vi "VR-Hall.vi"(8 "error in (no error)":errorcluster, 11 "Node Ptr":T2 format="%.0x") -> (0 "error out":errorcluster)   [LabVIEW 2016, in "DCM System Explorer.lvlib"]
uses:
  DCM System Explorer.lvlib
  <vilib>/NI Veristand/Custom Device API/Custom Device Item Ref.ctl
  <vilib>/Powertrain Controls/Device Drivers/VR-Hall/RevC/Real-Time/Support/Vr_Hall_mode_control_revc.ctl
  Shared/DCM Properties.vi
  <vilib>/NI Veristand/Custom Device API/Get Item Property (Double Array).vi
  <vilib>/NI Veristand/Custom Device API/Set Item Property (Double Array).vi
  <vilib>/NI VeriStand/Custom Device API/Custom Device API.lvlib
  DCM Shared.lvlib
panel:
  out "Channel":string[](array[string])=["Channel 1", "Channel 2", "Channel 3", "Channel 4", "Channel 5"]
  in  "Arming Threshold [V]":dbl[](array[numeric])
  in  "VR-Hall Mode Select":T1[](array[typedef])
  in  "Header":cluster{"Section Name":string}={"Section Name"="VR-Hall Initial Settings"}
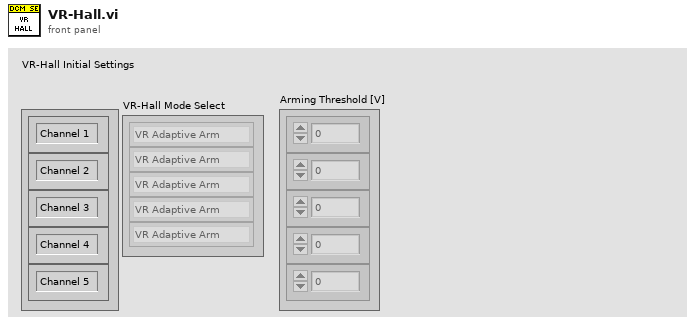
[diagram p1: front panel]
types:
  T1 = typedef "Vr_Hall_mode_control_revc.ctl" = enum32{"VR Adaptive Arm", "VR Manual Arm", "Hall", "Hall w/ Pull-up"}
  T2 = typedef "Custom Device API.lvlib/Custom Device Item Ref.ctl" = u64
  T3 = typedef "Custom Device API.lvlib/Custom Device Commands.ctl" = enum16{"Default", "Item renamed", "Shutdown", "Dynamic button pressed"}
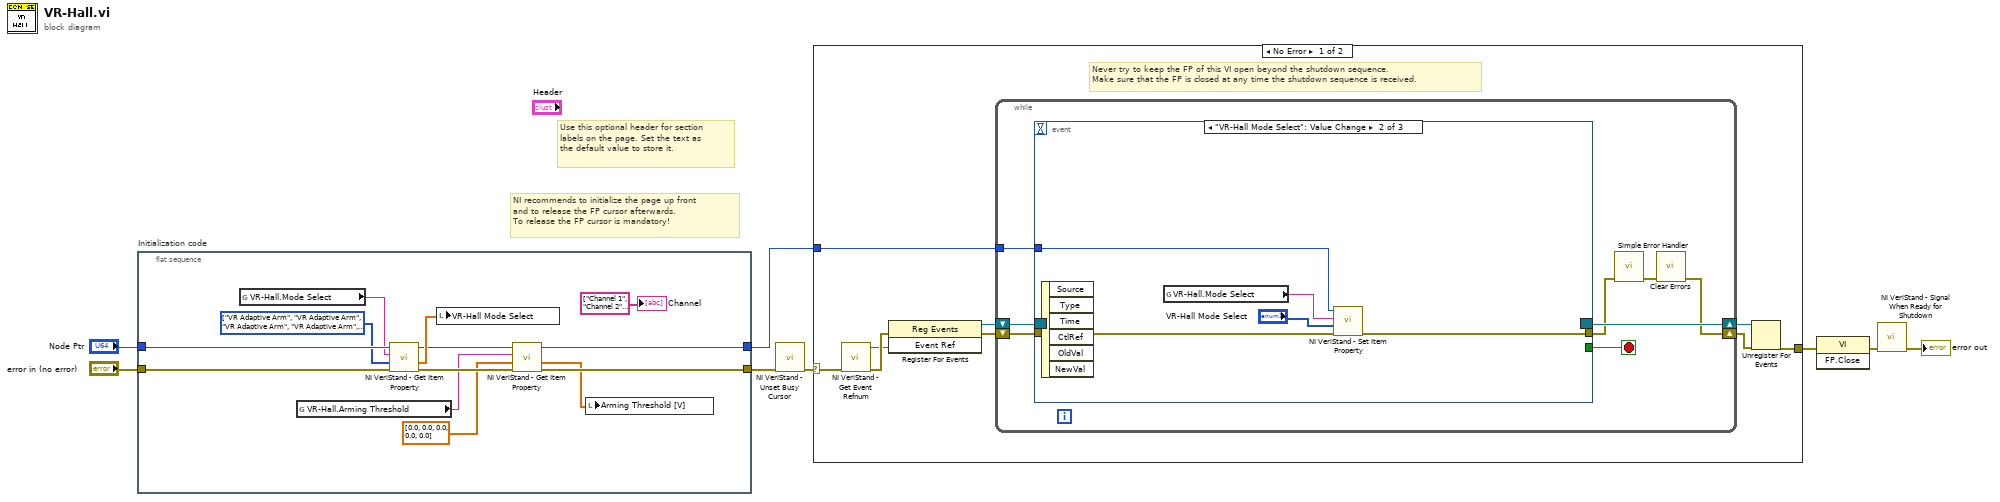
[diagram p0: block diagram]
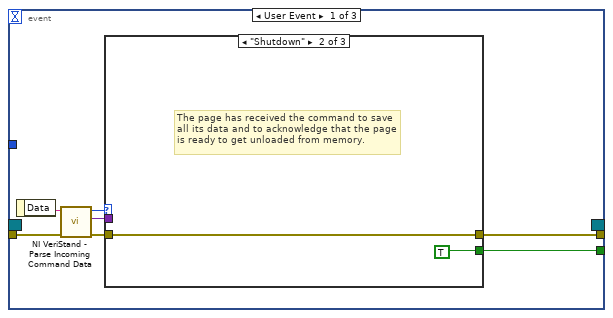
[diagram p2: hidden frame]
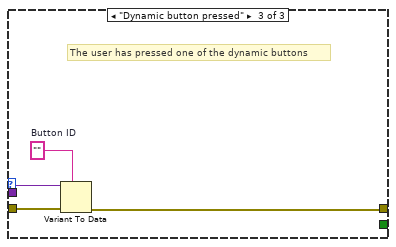
[diagram p4: hidden frame]
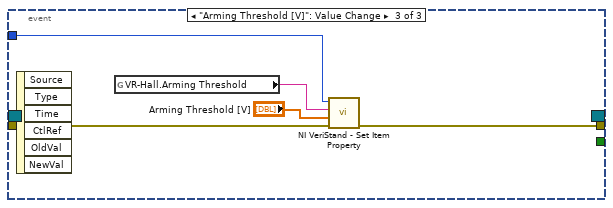
[diagram p5: hidden frame]
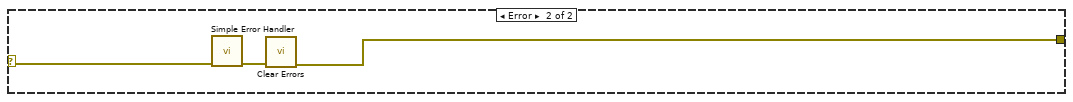
[diagram p6: hidden frame]
diagram:
  # "Use this optional header for section labels on the page. Set the text as the default value to store it."
  # "NI recommends to initialize the page up front\nand to release the FP cursor afterwards.\nTo release the FP cursor is mandatory!"
  n1 = flat-sequence "Initialization code" {
    tunnel: "error in (no error)" -> [w19]
    tunnel: "Node Ptr" -> [w20]
    tunnel: [w13] -> w4
    tunnel: [w14] -> w1
    frame #0 {
      w17 = T1[] [enum."VR Adaptive Arm", enum."VR Adaptive Arm", enum."VR Adaptive Arm", enum."VR Adaptive Arm", enum."VR Adaptive Arm"] items=["VR Adaptive Arm", "VR Manual Arm", "Hall", "Hall w/ Pull-up"] ("VR-Hall Mode Select")
      n2 = global read "DCM Properties.vi" "VR-Hall.Mode Select"() -> (w18:string)
      n3 = global read "DCM Properties.vi" "VR-Hall.Arming Threshold"() -> (w11:string)
      n4 = call-poly <vilib>:"NI VeriStand - Get Item Property.vi"("error in (no error)"=w19, "Default Value"=w17, "Property Name"=w18, "Item Ref in"=w20) -> ("error out"=w12:errorcluster, "Value"=w16:dbl[], "Item Ref out"=w15:T2)  [unwired: 4 in, 1 out]
      n5 = local write "VR-Hall Mode Select"(w16) -> ()
      n6 = call-poly <vilib>:"NI VeriStand - Get Item Property.vi"("error in (no error)"=w12, "Default Value"=dbl[] [0.0, 0.0, 0.0, 0.0, 0.0] ("Arming Threshold [V]"), "Property Name"=w11, "Item Ref in"=w15) -> ("error out"=w13:errorcluster, "Value"=w9:dbl[], "Item Ref out"=w14:T2)  [unwired: 4 in, 1 out]
      n7 = local write "Arming Threshold [V]"(w9) -> ()
      "Channel" <- string[] ["Channel 1", "Channel 2", "Channel 3", "Channel 4", "Channel 5"] ("Channel")
    }
  }
  n8 = call <vilib>:"NI VeriStand - Unset Busy Cursor.vi"("error in (no error)"=w4) -> ("error out"=w3:errorcluster)  [unwired: 10 out]
  n9 = case shown="No Error" w3 {
    selector: w3 -> [w22 w65]
    tunnel: [w27 w63] -> w8
    tunnel: w1 -> [w23 _]
    frame No Error {
      # "Never try to keep the FP of this VI open beyond the shutdown sequence.\nMake sure that the FP is closed at any time the shutdown sequence is received."
      n10 = call <vilib>:"NI VeriStand - Get Event Refnum.vi"("error in (no error)"=w22) -> ("error out"=w30:errorcluster, "Event Ref"=w26:refnum<user-event>)  [unwired: 9 out]
      n11 = register-events(error in=w30, w26) -> (reference out=w24:refnum<event-registration>, error out=w25:errorcluster)  [unwired: 1 in]
      n12 = while {
        tunnel: w23 -> [w34]
        shift-right: [w31] -> w28
        shift-left: w25 -> [w37]
        shift-right: [w38] -> w29
        shift-left: w24 -> [w36]
        stop <- w35 stop-if-true
        n13 = event shown="[1] \"VR-Hall Mode Select\": Value Change" {
          selector: w36 -> [_ _ _]
          dyn-events: [_ _ _] -> w38
          timeout: _ -> [_ _ _]
          tunnel: w37 -> [w45 w57 w62]
          tunnel: [w41 _ _] -> w35
          tunnel: [w40 w56 w61] -> w33
          tunnel: w34 -> [_ w54 w58]
          event User Event {
            n14 = event-data() -> ("Data"=w44:string)  [unwired: 1 out]
            n15 = call <vilib>:"NI VeriStand - Parse Incoming Command Data.vi"("error in (no error)"=w45, "Incoming data"=w44) -> ("error out"=w43:errorcluster, "Outgoing data"=w39:variant, "Action"=w42:T3)  [unwired: 7 out]
            n16 = case shown="\"Shutdown\"" w42 {
              tunnel: w43 -> [w46 w47 w52]
              tunnel: [_ TRUE _] -> w41
              tunnel: [w46 w47 w49] -> w40
              tunnel: w39 -> [_ _ w51]
              frame "Default", Default {
              }
              frame "Shutdown" {
                # "The page has received the command to save all its data and to acknowledge that the page is ready to get unloaded from memory."
              }
              frame "Dynamic button pressed" {
                w50 = ""  # Button ID
                # "The user has pressed one of the dynamic buttons"
                n17 = Variant To Data(error in=w52, type=w50, Variant=w51) -> (error out=w49:errorcluster)  [unwired: 1 out]
              }
            }
          }
          event "VR-Hall Mode Select": Value Change {
            n18 = event-data() -> ()  [unwired: 7 out]
            n19 = global read "DCM Properties.vi" "VR-Hall.Mode Select"() -> (w55:string)
            n20 = call-poly <vilib>:"NI VeriStand - Set Item Property.vi"("error in (no error)"=w57, "Value"="VR-Hall Mode Select", "Property Name"=w55, "Item Ref in"=w54) -> ("error out"=w56:errorcluster)  [unwired: 5 in, 2 out]
          }
          event "Arming Threshold [V]": Value Change {
            n21 = event-data() -> ()  [unwired: 7 out]
            n22 = global read "DCM Properties.vi" "VR-Hall.Arming Threshold"() -> (w60:string)
            n23 = call-poly <vilib>:"NI VeriStand - Set Item Property.vi"("error in (no error)"=w62, "Value"="Arming Threshold [V]", "Property Name"=w60, "Item Ref in"=w58) -> ("error out"=w61:errorcluster)  [unwired: 5 in, 2 out]
          }
        }
        n24 = call <vilib>:"Simple Error Handler.vi"("error in (no error)"=w33) -> ("error out"=w32:errorcluster)  [unwired: 1 in, 7 out]
        n25 = call <vilib>:"Clear Errors.vi"("error in (no error)"=w32) -> ("error out"=w31:errorcluster)  [unwired: 1 in, 5 out]
      }
      n26 = Unregister For Events(event registration refnum=w29, error in=w28) -> (error out=w27:errorcluster)
    }
    frame Error {
      n27 = call <vilib>:"Simple Error Handler.vi"("error in (no error)"=w65) -> ("error out"=w64:errorcluster)  [unwired: 1 in, 7 out]
      n28 = call <vilib>:"Clear Errors.vi"("error in (no error)"=w64) -> ("error out"=w63:errorcluster)  [unwired: 1 in, 5 out]
    }
  }
  n29 = invoke class="VI" method="FP.Close"(error in=w8) -> (error out=w7:errorcluster)  [unwired: 2 in, 2 out]
  n30 = call <vilib>:"NI VeriStand - Signal When Ready for Shutdown.vi"("error in (no error)"=w7) -> ("error out"=→"error out":errorcluster)  [unwired: 10 out]
